vi "dummyPed.vi"(1 "file path (dialog if empty)":path, 5 "mask 1":i32[](array[numeric]), 7 "calo ch":i32, 9 "mask 2":i32[](array[numeric]), 11 "wcm ch":i32) -> (4 "ped 1":sgl[](array[numeric]), 6 "sigma 1":sgl[](array[numeric]), 8 "vcm ped":sgl, 10 "ped 2":sgl[](array[numeric]), 13 "caloped":sgl, 14 "calosigma":sgl, 15 "sigma 2":sgl[](array[numeric]))   [LabVIEW 2014]
uses:
  <vilib>/Utility/file.llb/Read From Spreadsheet File (DBL).vi
panel:
  out "all ped&sigma":sgl[](array[numeric])
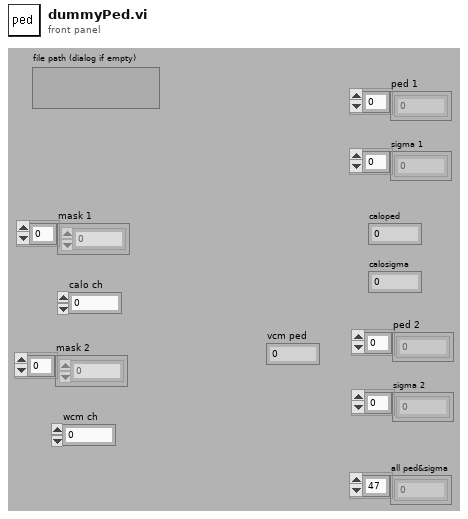
[diagram p1: front panel]
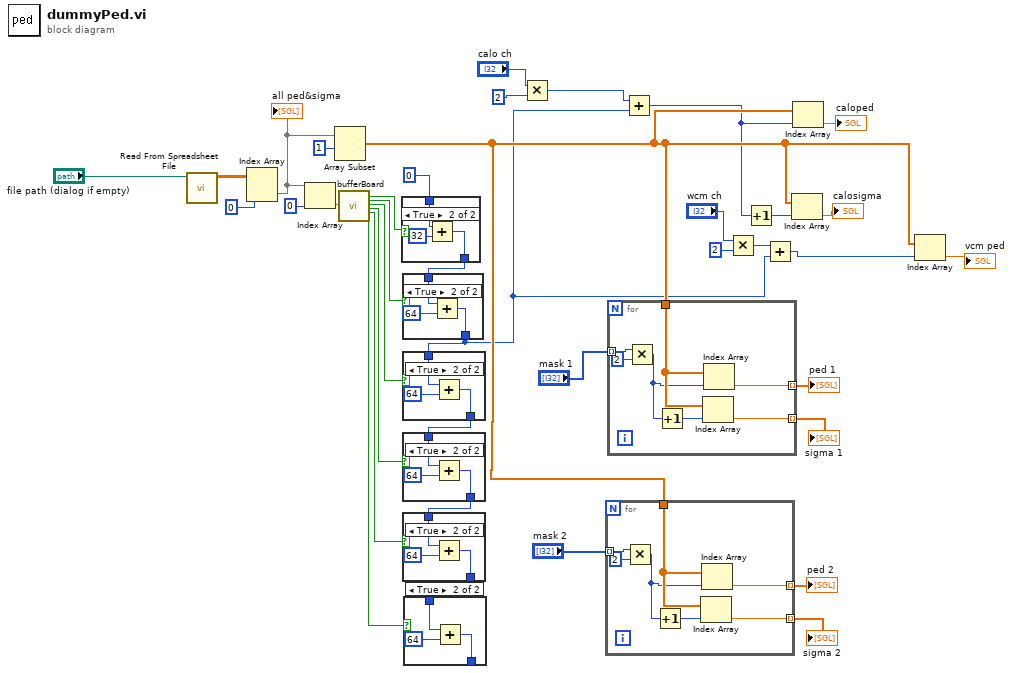
[diagram p0: block diagram]
diagram:
  n1 = call-poly <vilib>:"Read From Spreadsheet File.vi"("file path (dialog if empty)"="file path (dialog if empty)") -> ("all rows"=w37:dbl[][])  [unwired: 6 in, 4 out]
  n2 = Index Array(array=w37, index (col)=0 ("index (row)")) -> (element=w23:dbl[])  [unwired: 1 in]
  "all ped&sigma" <- w23
  n3 = Index Array(array=w23, index=0 ("length")) -> (element=w21:dbl)
  n4 = Array Subset(array=w23, index=1) -> (w25:dbl[])  [unwired: 1 in]
  n5 = call "bufferBoard.vi"(3:w21) -> ("peak"=w20:bool, "qdc1"=w18:bool, "qdc2"=w16:bool, "tdc1"=w15:bool, "qdc3"=w12:bool, "tdc2"=w11:bool)  [unwired: 19 in, 2 out]
  n6 = case shown="True" w20 {
    tunnel: 0 -> [w39 w42]
    tunnel: [w39 w40] -> w17
    frame False {
    }
    frame True {
      n7 = Add(x=w42, y=32) -> (x+y=w40:i32)
    }
  }
  n8 = case shown="True" w18 {
    tunnel: w17 -> [w43 w46]
    tunnel: [w43 w44] -> w1
    frame False {
    }
    frame True {
      n9 = Add(x=w46, y=64) -> (x+y=w44:i32)
    }
  }
  n10 = case shown="True" w16 {
    tunnel: w1 -> [w47 w50]
    tunnel: [w47 w48] -> w6
    frame False {
    }
    frame True {
      n11 = Add(x=w50, y=64) -> (x+y=w48:i32)
    }
  }
  n12 = case shown="True" w15 {
    tunnel: w6 -> [w51 w54]
    tunnel: [w51 w52] -> w14
    frame False {
    }
    frame True {
      n13 = Add(x=w54, y=64) -> (x+y=w52:i32)
    }
  }
  n14 = case shown="True" w12 {
    tunnel: w14 -> [w55 w58]
    tunnel: [w55 w56] -> w13
    frame False {
    }
    frame True {
      n15 = Add(x=w58, y=64) -> (x+y=w56:i32)
    }
  }
  n16 = case shown="True" w11 {
    tunnel: w13 -> [w59 w62]
    tunnel: [w59 w60] -> _
    frame False {
    }
    frame True {
      n17 = Add(x=w62, y=64) -> (x+y=w60:i32)
    }
  }
  n18 = Multiply(x="calo ch", y=2) -> (x*y=w8:i32)
  n19 = for {
    tunnel: "mask 2" -> [w65] mode=indexing
    tunnel: w25 -> [w68]
    tunnel: [w67] -> w28 mode=indexing
    tunnel: [w66] -> w27 mode=indexing
    n20 = Multiply(x=w65, y=2) -> (x*y=w64:i32)
    n21 = Increment(x=w64) -> (x+1=w69:i32)
    n22 = Index Array(array=w68, index=w69) -> (element=w66:dbl)
    n23 = Index Array(array=w68, index=w64) -> (element=w67:dbl)
  }
  "ped 2" <- w28
  "sigma 2" <- w27
  n24 = for {
    tunnel: "mask 1" -> [w72] mode=indexing
    tunnel: w25 -> [w75]
    tunnel: [w74] -> w31 mode=indexing
    tunnel: [w73] -> w30 mode=indexing
    n25 = Multiply(x=w72, y=2) -> (x*y=w71:i32)
    n26 = Increment(x=w71) -> (x+1=w76:i32)
    n27 = Index Array(array=w75, index=w76) -> (element=w73:dbl)
    n28 = Index Array(array=w75, index=w71) -> (element=w74:dbl)
  }
  "ped 1" <- w31
  "sigma 1" <- w30
  n29 = Add(x=w8, y=w1) -> (x+y=w7:i32)
  n30 = Multiply(x="wcm ch", y=2) -> (x*y=w3:i32)
  n31 = Increment(x=w7) -> (x+1=w33:i32)
  n32 = Add(x=w3, y=w1) -> (x+y=w2:i32)
  n33 = Index Array(array=w25, index=w33) -> (element=→"calosigma":dbl)
  n34 = Index Array(array=w25, index=w7) -> (element=→"caloped":dbl)
  n35 = Index Array(array=w25, index=w2) -> (element=→"vcm ped":dbl)
